vi "Create User Events.vi"(0 "Code String in":refnum<class "Code String.lvclass">, 11 "error in (no error)":errorcluster) -> (4 "Code String out":refnum<class "Code String.lvclass">, 15 "error out":errorcluster)   [LabVIEW 2016, in "Code String.lvclass"]
doc: "Creates references for the User Events used to communicate with the Code String.\n--------------------\nCopyright (c) 2019 Analog Devices, Inc. All rights reserved.\n\nRedistribution and use in source and binary forms, with or without modification,\nare permitted provided that the following conditions are met:\n - Redistributions of source code must retain the above copyright notice, this\n list of conditions and the following disclaimer.\n - Redistributions in binary form must reproduce the above copyright notice,\n this list of conditions and the following disclaimer in the documentation\n and/or other materials provided with the distribution.\n - Modified versions of the software must be conspicuously marked as such.\n - This software is licensed solely and exclusively for use with\n processors/products manufactured by or for Analog Devices, Inc.\n - This software may not be combined or merged with other code in any manner\n that would cause the software to become subject to terms and conditions\n which differ from those listed here.\n - Neither the name of Analog Devices, Inc. nor the names of its contributors\n may be used to endorse or promote products derived from this software\n without specific prior written permission.\n - The use of this software may or may not infringe the patent rights of one or\n more patent holders. This license does not release you from the requirement\n that you obtain separate licenses from these patent holders to use this\n software.\n\nTHIS SOFTWARE IS PROVIDED BY ANALOG DEVICES, INC. AND CONTRIBUTORS \"AS IS\" AND\nANY EXPRESS OR IMPLIED WARRANTIES, INCLUDING, BUT NOT LIMITED TO,\nNON-INFRINGEMENT, TITLE, MERCHANTABILITY AND FITNESS FOR A PARTICULAR PURPOSE\nARE DISCLAIMED. IN NO EVENT SHALL ANALOG DEVICES, INC. OR CONTRIBUTORS BE LIABLE\nFOR ANY DIRECT, INDIRECT, INCIDENTAL, SPECIAL, EXEMPLARY, PUNITIVE OR\nCONSEQUENTIAL DAMAGES (INCLUDING, BUT NOT LIMITED TO, DAMAGES ARISING OUT OF\nCLAIMS OF INTELLECTUAL PROPERTY RIGHTS INFRINGEMENT; PROCUREMENT OF SUBSTITUTE\nGOODS OR SERVICES; LOSS OF USE, DATA, OR PROFITS; OR BUSINESS INTERRUPTION)\nHOWEVER CAUSED AND ON ANY THEORY OF LIABILITY, WHETHER IN CONTRACT, STRICT\nLIABILITY, OR TORT (INCLUDING NEGLIGENCE OR OTHERWISE) ARISING IN ANY WAY OUT OF\nTHE USE OF THIS SOFTWARE, EVEN IF ADVISED OF THE POSSIBILITY OF SUCH DAMAGE.\n\n2019-01-10-7CBSD SLA"
uses:
  Code String.lvclass
  Menu Item.ctl
  Code String.lvclass/Code String.ctl
panel:
  # "Copyright (c) 2019 Analog Devices, Inc.  All rights reserved.\n\nRedistribution and use in source and binary forms, with or without modification,\nare permitted provided that the following conditions are met:\n  - Redistributions of source code must retain the above copyright notice, this\n    list of conditions and the following disclaimer.\n  - Redistributions in binary form must reproduce the above copyright notice,\n    this list of conditions and the following disclaimer in the documentation\n    and/or other materials provided with the distribution.\n  - Modified versions of the software must be conspicuously marked as such.\n  - This software is licensed solely and exclusively for use with\n    processors/products manufactured by or for Analog Devices, Inc.\n  - This software may not be combined or merged with other code in any manner\n    that would cause the software to become subject to terms and conditions\n    which differ from those listed here.\n  - Neither the name of Analog Devices, Inc. nor the names of its contributors\n    may be used to endorse or promote products derived from this software\n    without specific prior written permission.\n  - The use of this software may or may not infringe the patent rights of one or\n    more patent holders.  This license does not release you from the requirement\n    that you obtain separate licenses from these patent holders to use this\n    software.\n\nTHIS SOFTWARE IS PROVIDED BY ANALOG DEVICES, INC. AND CONTRIBUTORS \"AS IS\" AND\nANY EXPRESS OR IMPLIED WARRANTIES, INCLUDING, BUT NOT LIMITED TO,\nNON-INFRINGEMENT, TITLE, MERCHANTABILITY AND FITNESS FOR A PARTICULAR PURPOSE\nARE DISCLAIMED. IN NO EVENT SHALL ANALOG DEVICES, INC. OR CONTRIBUTORS BE LIABLE\nFOR ANY DIRECT, INDIRECT, INCIDENTAL, SPECIAL, EXEMPLARY, PUNITIVE OR\nCONSEQUENTIAL DAMAGES (INCLUDING, BUT NOT LIMITED TO, DAMAGES ARISING OUT OF\nCLAIMS OF INTELLECTUAL PROPERTY RIGHTS INFRINGEMENT; PROCUREMENT OF SUBSTITUTE\nGOODS OR SERVICES; LOSS OF USE, DATA, OR PROFITS; OR BUSINESS INTERRUPTION)\nHOWEVER CAUSED AND ON ANY THEORY OF LIABILITY, WHETHER IN CONTRACT, STRICT\nLIABILITY, OR TORT (INCLUDING NEGLIGENCE OR OTHERWISE) ARISING IN ANY WAY OUT OF\nTHE USE OF THIS SOFTWARE, EVEN IF ADVISED OF THE POSSIBILITY OF SUCH DAMAGE.\n\n2019-01-10-7CBSD SLA"
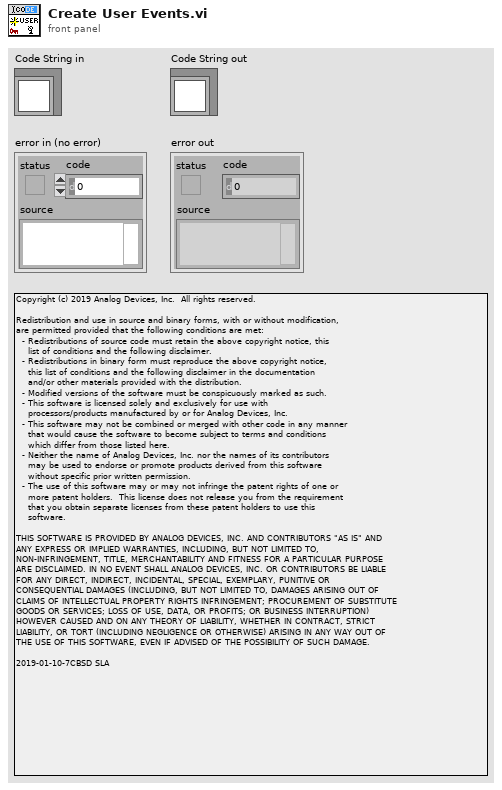
[diagram p1: front panel]
types:
  T1 = typedef "Code String.lvclass/Menu Item.ctl" = cluster{"Item Path":string, "Visible?":bool, "Checked?":bool}
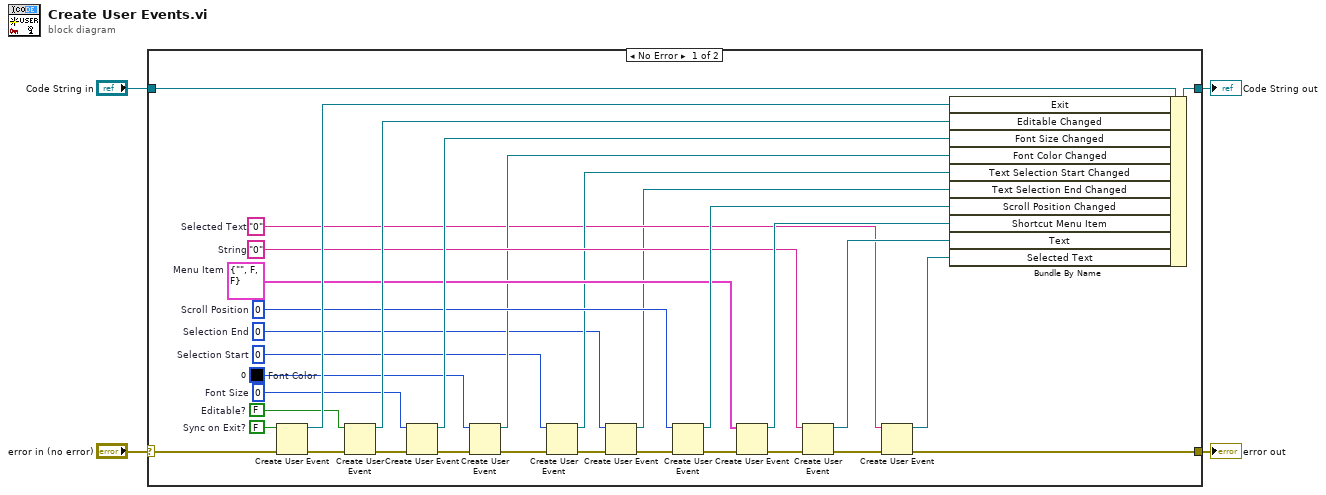
[diagram p0: block diagram]
diagram:
  n1 = case shown="No Error" "error in (no error)" {
    selector: "error in (no error)" -> [w35 w38]
    tunnel: [w9 w38] -> w3
    tunnel: [w33 w37] -> w1
    tunnel: "Code String in" -> [w36 w37]
    frame No Error {
      w8 = u32 0  # Selection Start
      w6 = u32 0  # Selection End
      w11 = "0"  # Selected Text
      w16 = u32 0  # Font Color
      w18 = "0"  # String
      w23 = T1 {"Item Path"="", "Visible?"=FALSE, "Checked?"=FALSE}  # Menu Item
      w25 = u32 0  # Scroll Position
      w27 = u32 0  # Font Size
      w29 = FALSE  # Editable?
      w34 = FALSE  # Sync on Exit?
      n2 = Create User Event(user event datatype=w34, error in=w35) -> (user event=w32:refnum<user-event>, error out=w31:errorcluster)
      n3 = Create User Event(user event datatype=w29, error in=w31) -> (user event=w30:refnum<user-event>, error out=w28:errorcluster)
      n4 = Create User Event(user event datatype=w27, error in=w28) -> (user event=w26:refnum<user-event>, error out=w17:errorcluster)
      n5 = Create User Event(user event datatype=w16, error in=w17) -> (user event=w15:refnum<user-event>, error out=w14:errorcluster)
      n6 = Create User Event(user event datatype=w8) -> (user event=w13:refnum<user-event>)  [unwired: 1 in, 1 out]
      n7 = Create User Event(user event datatype=w6, error in=w14) -> (user event=w5:refnum<user-event>, error out=w7:errorcluster)
      n8 = Create User Event(user event datatype=w25, error in=w7) -> (user event=w24:refnum<user-event>, error out=w21:errorcluster)
      n9 = Create User Event(user event datatype=w23, error in=w21) -> (user event=w22:refnum<user-event>, error out=w20:errorcluster)
      n10 = Create User Event(user event datatype=w18, error in=w20) -> (user event=w19:refnum<user-event>, error out=w10:errorcluster)
      n11 = Create User Event(user event datatype=w11, error in=w10) -> (user event=w12:refnum<user-event>, error out=w9:errorcluster)
      n12 = Bundle By Name(cluster=w36, "Exit"=w32, "Editable Changed"=w30, "Font Size Changed"=w26, "Font Color Changed"=w15, "Text Selection Start Changed"=w13, "Text Selection End Changed"=w5, "Scroll Position Changed"=w24, "Shortcut Menu Item"=w22, "Text"=w19, "Selected Text"=w12) -> (w33:refnum<class "Code String.lvclass">)
    }
    frame Error {
    }
  }
  "error out" <- w3
  "Code String out" <- w1
